vi "SM_VDUT ON-OFF.vi"(2 "error in (no error)":errorcluster, 3 "Port2 IN":u8 format="%x", 4 "Power State":enum16{"Vdut On", "Vdut Off"}(ring)) -> (0 "error out":errorcluster, 1 "Port2 OUT":u8 format="%x")   [LabVIEW 2011]
doc: "This VI will turn ON or OFF the VDUT power supply by changing Port2 bit 1."
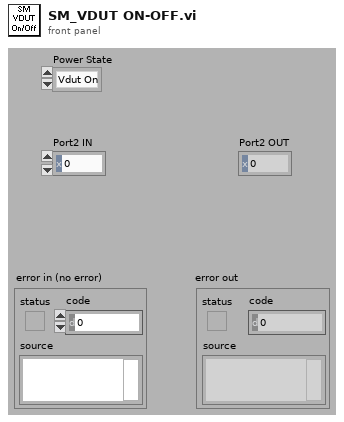
[diagram p1: front panel]
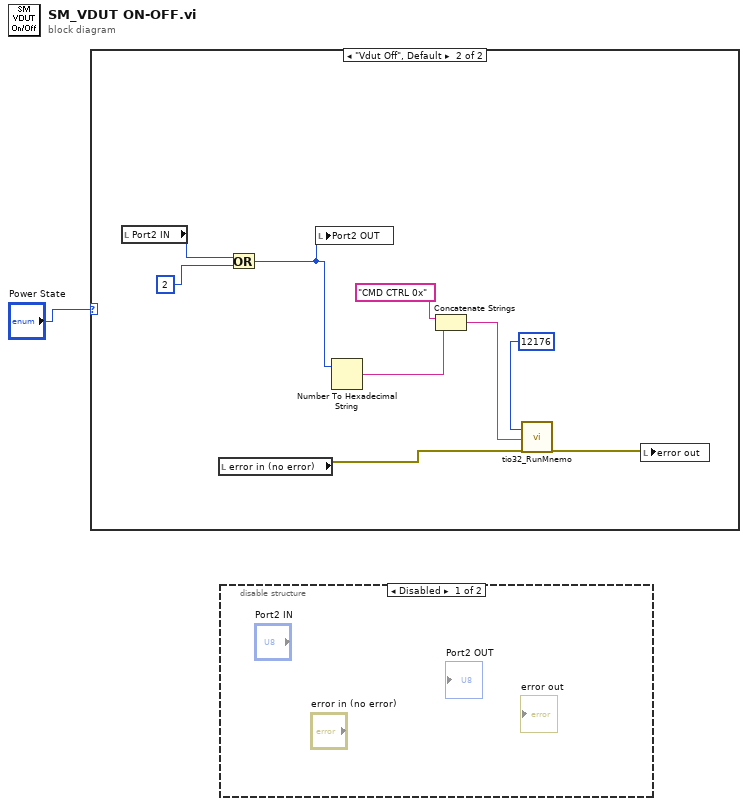
[diagram p0: block diagram]
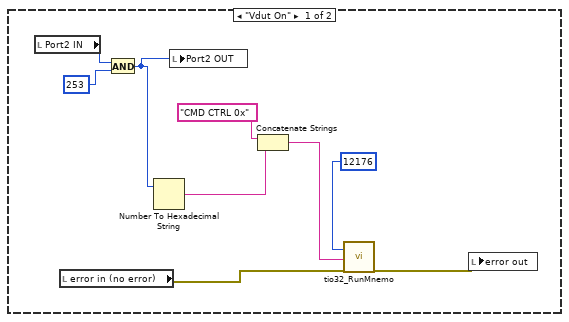
[diagram p3: hidden frame]
diagram:
  n1 = case shown="\"Vdut Off\", Default" "Power State" {
    frame "Vdut On" {
      n2 = local read "Port2 IN"() -> (w5:u8)
      n3 = local read "error in (no error)"() -> (w2:errorcluster)
      n4 = And(x=w5, y=u8 253) -> (x .and. y?=w4:u8)
      n5 = Number To Hexadecimal String(2:w4) -> (0:w6:string)  [unwired: 1 in]
      n6 = local write "Port2 OUT"(w4) -> ()
      n7 = Concatenate Strings("CMD CTRL 0x" ("command string"), w6) -> (w7:string)
      n8 = call "tio32_RunMnemo.vi"("Device address"=12176, "command string"=w7, "error in (no error)"=w2) -> ("error out"=w3:errorcluster)  [unwired: 6 in, 10 out]
      n9 = local write "error out"(w3) -> ()
    }
    frame "Vdut Off", Default {
      n10 = local read "Port2 IN"() -> (w15:u8)
      n11 = local read "error in (no error)"() -> (w11:errorcluster)
      n12 = Or(x=w15, y=u8 2) -> (x .or. y?=w13:u8)
      n13 = local write "Port2 OUT"(w13) -> ()
      n14 = Number To Hexadecimal String(2:w13) -> (0:w16:string)  [unwired: 1 in]
      n15 = Concatenate Strings("CMD CTRL 0x" ("command string"), w16) -> (w17:string)
      n16 = call "tio32_RunMnemo.vi"("Device address"=12176, "command string"=w17, "error in (no error)"=w11) -> ("error out"=w12:errorcluster)  [unwired: 6 in, 10 out]
      n17 = local write "error out"(w12) -> ()
    }
  }
  n18 = disable-structure shown="Disabled" {
    frame Disabled {
    }
    frame Enabled {
    }
  }
